vi "Joystick Analyze.vi"(2 "Joystick Name":T1) -> (3 "Slow Drive Enabled?":bool, 4 "Stabilize Gain":dbl, 5 "ResetGyro":bool, 6 "x":dbl, 7 "y":dbl, 8 "Open Jack":bool, 9 "Stabilize":bool, 10 "Close Jack":bool)   [LabVIEW 2011]
uses:
  <vilib>/Rock Robotics/WPI/Joystick/WPI_JoystickDevRef.ctl
  <vilib>/Rock Robotics/WPI/Joystick/WPI_JoystickDeviceEnum.ctl
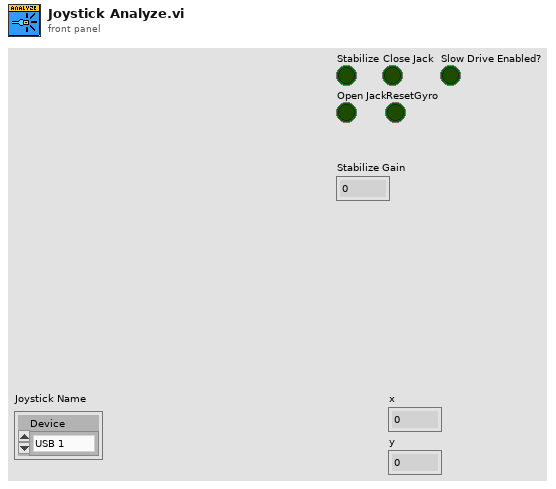
[diagram p1: front panel]
types:
  T1 = typedef "WPI_JoystickDevRef.ctl" = cluster{"Device":T2}
  T2 = typedef "WPI_JoystickDeviceEnum.ctl" = enum16{"USB 1", "USB 2", "USB 3", "USB 4", "Kinect 1", "Kinect 2"}
  T3 = typedef "WPI_JoystickButtonState.ctl" = cluster{"Button 1":bool, "Button 2":bool, "Button 3":bool, "Button 4":bool, "Button 5":bool, "Button 6":bool, "Button 7":bool, "Button 8":bool, "Button 9":bool, "Button 10":bool, "Button 11":bool, "Button 12":bool}
  T4 = cluster{"axis 1 (x)":dbl, "axis 2 (y)":dbl, "axis 3 (throttle)":dbl, "axis 4":dbl, "axis 5":dbl, "axis 6":dbl}
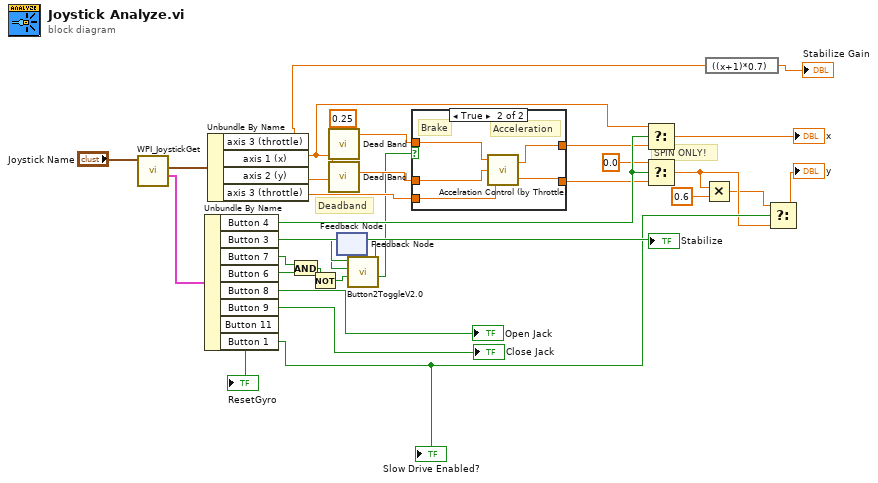
[diagram p0: block diagram]
diagram:
  w30 = 0.25 ("Dead Band")
  # "Deadband"
  # "SPIN ONLY!"
  n1 = call <vilib>:"WPI_JoystickGet.vi"("JoystickDevRef"="Joystick Name") -> ("Buttons"=w33:T3, "Axes"=w34:T4)  [unwired: 1 in, 4 out]
  n2 = Unbundle By Name(w33) -> ("Button 4"=w29:bool, "Button 3"=→"Stabilize":bool, "Button 7"=w16:bool, "Button 6"=w15:bool, "Button 8"=→"Open Jack":bool, "Button 9"=→"Close Jack":bool, "Button 11"=→"ResetGyro":bool, "Button 1"=w5:bool)
  "Slow Drive Enabled?" <- w5
  n3 = Unbundle By Name(w34) -> ("axis 3 (throttle)"=w13:dbl, "axis 1 (x)"=w20:dbl, "axis 2 (y)"=w31:dbl, "axis 3 (throttle)"=w23:dbl)
  n4 = And(x=w16, y=w15) -> (x .and. y?=w7:bool)
  n5 = Not(x=w7) -> (.not. x?=w6:bool)
  n6 = call "Dead Band.vi"("Axis In"=w20, "Dead Band"=w30) -> ("Axis Out"=w25:dbl)  [unwired: 9 in]
  n7 = call "Dead Band.vi"("Axis In"=w31, "Dead Band"=w30) -> ("Axis Out"=w24:dbl)  [unwired: 9 in]
  n8 = feedback #1() -> (w9:bool)  [unwired: 1 in]
  n9 = feedback #2() -> (w11:bool)  [unwired: 1 in]
  n10 = call "Button2ToggleV2.0.vi"("a"=w6, "fNodeA(in)"=w9, "fNodeB"=w11) -> ("Result(clone)"=w8:bool, "fNodeA(out)"=w10:bool, "Latched Bool (+fNodeB)"=w12:bool)  [unwired: 6 in]
  n11 = feedback-in #1(w10) -> ()
  n12 = feedback-in #2(w12) -> ()
  n13 = case shown="True" w8 {
    tunnel: w25 -> [w36 w38]
    tunnel: w24 -> [w35 w39]
    tunnel: w23 -> [_ w37]
    tunnel: [w36 w41] -> w22
    tunnel: [w35 w40] -> w21
    frame False {
    }
    frame True {
      # "Brake"
      # "Acceleration"
      n14 = call "Accelration Control (by Throttle).vi"("acc"=w37, "Yinput"=w39, "Xinput"=w38) -> ("Youtput"=w40:dbl, "Xoutput"=w41:dbl)
    }
  }
  n15 = Select(t=w20, s=w29, f=w22) -> (s? t:f=→"x":dbl)
  n16 = Select(t=0.0, s=w29, f=w21) -> (s? t:f=w3:dbl)
  n17 = Multiply(x=w3, y=0.6) -> (x*y=w2:dbl)
  n18 = expression code="((x+1)*0.7)"(w13) -> (→"Stabilize Gain":dbl)
  n19 = Select(t=w2, s=w5, f=w3) -> (s? t:f=→"y":dbl)
